vi "DIALOG_Bundle Magic Init.vi"(10 "Why are we here?":T1, 11 "Stationary VI Ref":refnum<vi>) -> ()   [LabVIEW 2023]
panel:
  out "Title":string
  out "Prog Msg 1":string
  out "Prog Msg 2":string
  out "Horizontal Pointer Slide":u32(slide) caption="Progress Bar" max=295 step=1 scale=0.0..295.0
  out "Main Msg":string
  out "error out":errorcluster
  in  "error in (no error)":errorcluster
  in  "Close":bool
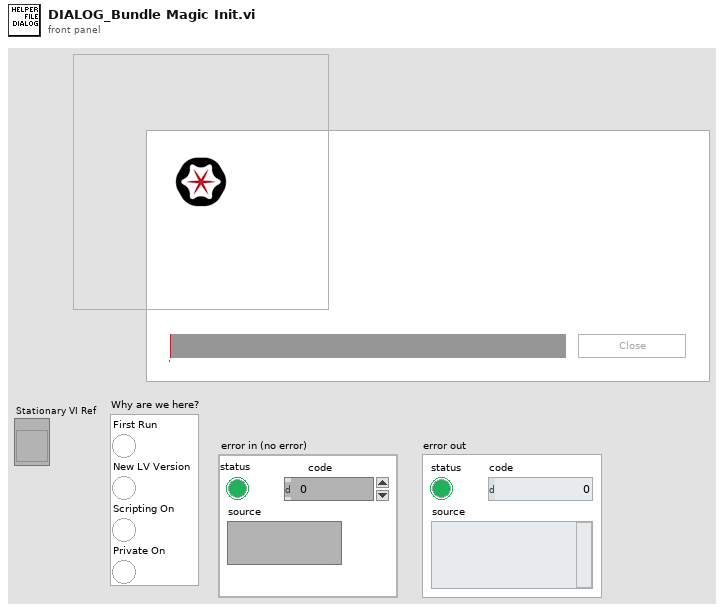
[diagram p1: front panel]
types:
  T1 = cluster{"First Run":bool, "New LV Version":bool, "Scripting On":bool, "Private On":bool}
  T2 = cluster{"Done":refnum<user-event>, "Msg 1":refnum<user-event>, "Msg 2":refnum<user-event>, "Prog Max":refnum<user-event>, "Prog Ct":refnum<user-event>}
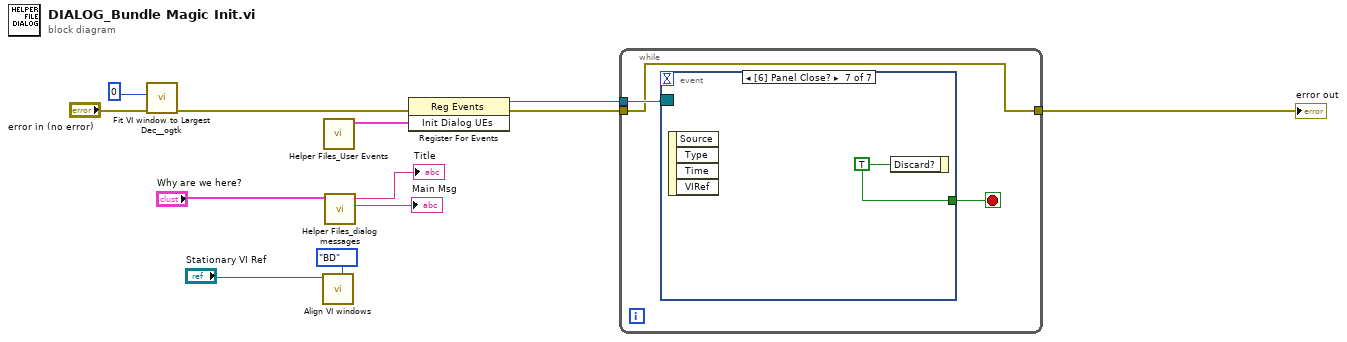
[diagram p0: block diagram]
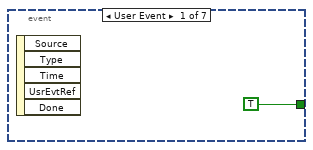
[diagram p2: hidden frame]
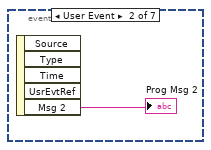
[diagram p3: hidden frame]
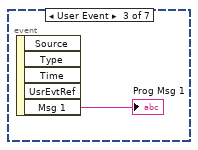
[diagram p4: hidden frame]
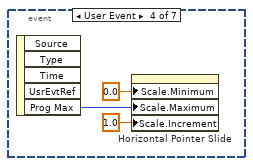
[diagram p5: hidden frame]
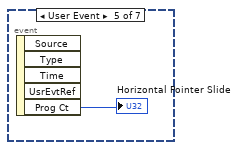
[diagram p6: hidden frame]
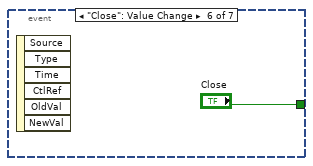
[diagram p7: hidden frame]
diagram:
  n1 = call <userlib>:"Fit VI window to Largest Dec__ogtk.vi"("error in (no error)"="error in (no error)", "border spacing (2 px)"=0) -> ("error out"=w11:errorcluster)  [unwired: 4 in, 1 out]
  n2 = call "Align VI windows.vi"("Align to"=enum16{"FP", "BD"}."BD", "Stationary VI Ref"="Stationary VI Ref") -> ()  [unwired: 9 in, 1 out]
  n3 = call "Helper Files_User Events.vi"() -> ("Init Dialog UEs"=w7:T2)  [unwired: 11 in]
  n4 = call "Helper Files_dialog messages.vi"("Why are we here?"="Why are we here?") -> ("Main Msg"=→"Main Msg":string, "Title Message"=→"Title":string)  [unwired: 9 in]
  n5 = register-events(error in=w11, w7) -> (reference out=w12:refnum<event-registration>, error out=w9:errorcluster)  [unwired: 1 in]
  n6 = while {
    tunnel: w12 -> [w15]
    tunnel: w9 -> [w13]
    tunnel: [w13] -> w8
    stop <- w14 stop-if-true
    n7 = event shown="[6] Panel Close?" {
      selector: w15 -> [_ _ _ _ _ _ _]
      dyn-events: _ -> [_ _ _ _ _ _ _]
      timeout: _ -> [_ _ _ _ _ _ _]
      tunnel: [TRUE _ _ _ _ "Close" w24] -> w14
      event User Event {
        n8 = event-data() -> ()  [unwired: 1 in, 5 out]
      }
      event User Event {
        n9 = event-data() -> ("Msg 2"=→"Prog Msg 2":string)  [unwired: 1 in, 4 out]
      }
      event User Event {
        n10 = event-data() -> ("Msg 1"=→"Prog Msg 1":string)  [unwired: 1 in, 4 out]
      }
      event User Event {
        n11 = event-data() -> ("Prog Max"=w21:u32)  [unwired: 1 in, 4 out]
        n12 = property on="Horizontal Pointer Slide" class="Slide (strict)"("Scale.Minimum"=0.0 ("Data Entry Limits:Minimum"), "Scale.Maximum"=w21, "Scale.Increment"=1.0 ("Data Entry Limits:Increment")) -> ()  [unwired: 2 in, 2 out]
      }
      event User Event {
        n13 = event-data() -> ("Prog Ct"=→"Horizontal Pointer Slide":u32)  [unwired: 1 in, 4 out]
      }
      event "Close": Value Change {
        n14 = event-data() -> ()  [unwired: 1 in, 6 out]
      }
      event Panel Close? {
        w24 = TRUE ("Discard?")
        n15 = event-data() -> ()  [unwired: 1 in, 4 out]
        n16 = event-data("Discard?"=w24) -> ()  [unwired: 1 in, 1 out]
      }
    }
  }
  "error out" <- w8
